vi "write_to_file_test.vi"(6 "freq":dbl[](array[numeric]), 7 "name or relative path":path, 8 "ua":dbl[](array[numeric]), 9 "count":dbl[](array[numeric]), 10 "osc":dbl[](array[numeric]), 11 "n":dbl[](array[numeric])) -> ()   [LabVIEW 2022 SP3]
panel:
  out "concatenated string":string
  out "spreadsheet string":string
  out "?":dbl[][](array[numeric])
  # "output_text_file_3.txt"
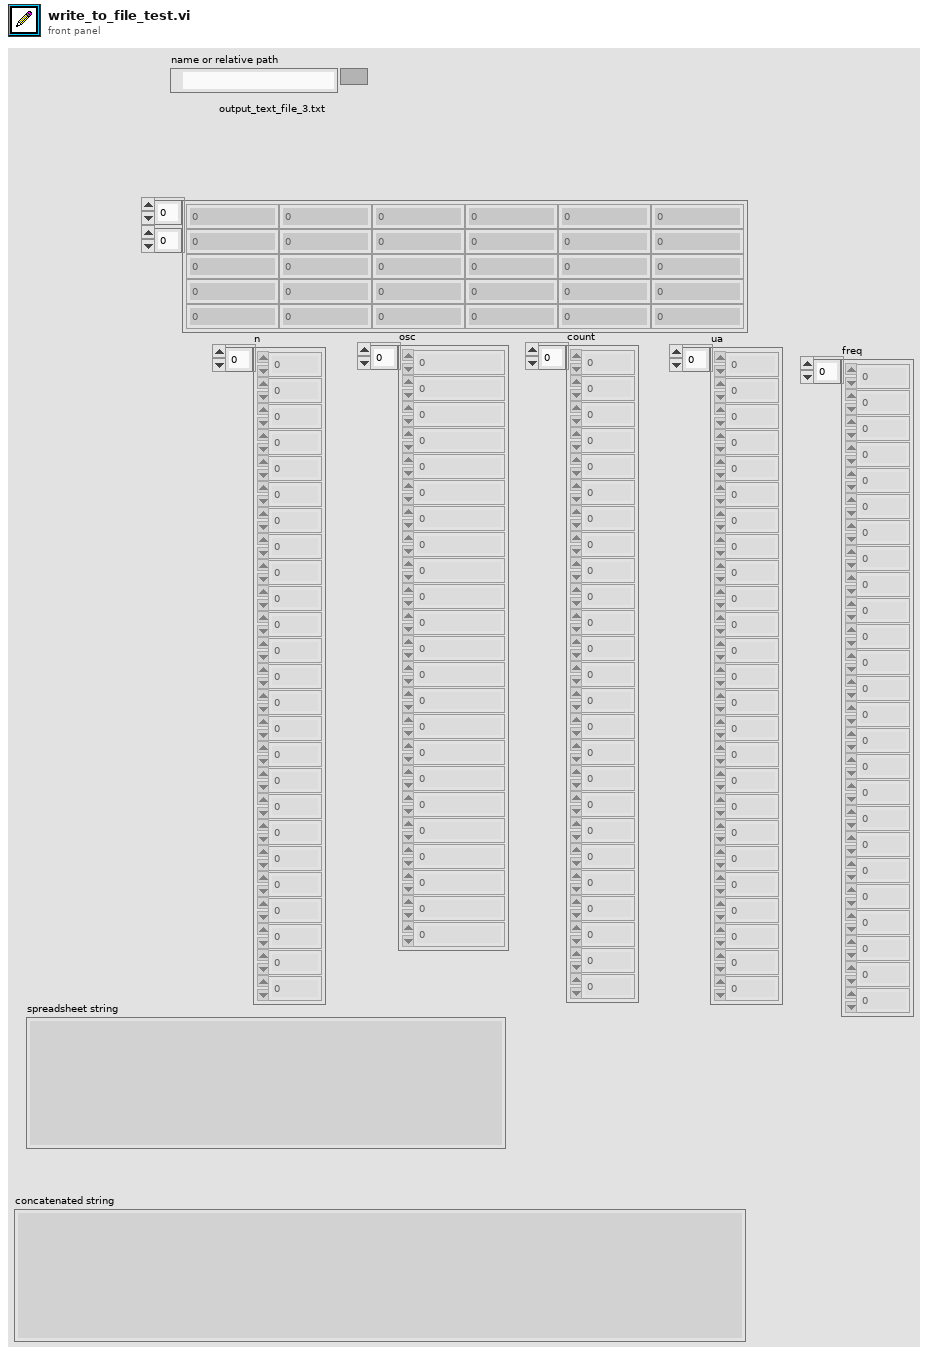
[diagram p1: front panel]
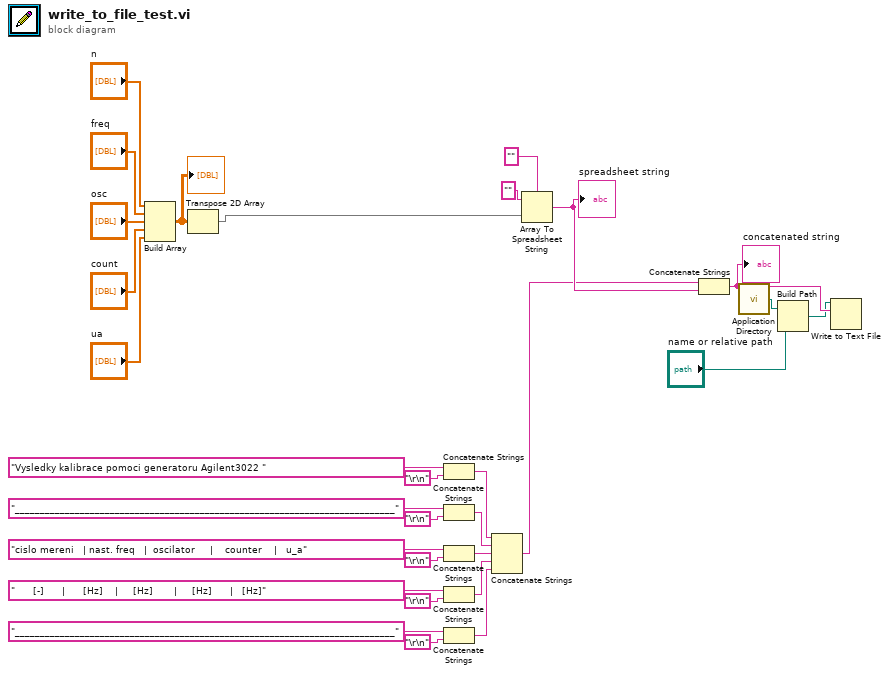
[diagram p0: block diagram]
diagram:
  n1 = Build Array("n", "freq", "osc", "count", "ua") -> (w15:dbl[][])
  "?" <- w15
  n2 = Transpose 2D Array(2D array=w15) -> (transposed array=w14:dbl[][])
  n3 = Concatenate Strings("Vysledky kalibrace pomoci generatoru Agilent3022 " ("String"), "\r\n") -> (w2:string)
  n4 = Concatenate Strings("____________________________________________________________________________" ("String"), "\r\n") -> (w9:string)
  n5 = Concatenate Strings("cislo mereni   | nast. freq   |  oscilator     |    counter    |   u_a" ("String"), "\r\n") -> (w8:string)
  n6 = Concatenate Strings("      [-]      |      [Hz]    |     [Hz]       |     [Hz]      |   [Hz]" ("String"), "\r\n") -> (w7:string)
  n7 = Concatenate Strings("____________________________________________________________________________" ("String"), "\r\n") -> (w6:string)
  n8 = Concatenate Strings(w2, w9, w8, w7, w6) -> (w5:string)
  n9 = Array To Spreadsheet String(delimiter (Tab)="", array=w14, 3:"" ("format string")) -> (spreadsheet string=w23:string)
  "spreadsheet string" <- w23
  n10 = Concatenate Strings(w5, w23) -> (w21:string)
  "concatenated string" <- w21
  n11 = call <vilib>:"Application Directory.vi"() -> ("Application Directory"=w22:path)
  n12 = Build Path(base path=w22, name or relative path="name or relative path") -> (appended path=w20:path)
  n13 = Write to Text File(file (use dialog)=w20, text=w21) -> ()  [unwired: 2 in, 3 out]
